vi "FipsAdjacent.vi"() -> (11 "Fips":i32[](array[numeric]))   [LabVIEW 2017] (continued)
TX\"\t48359\t\"Quay County, NM\"\t35037\n\"Oldham County, TX\"\t48359\t\"Deaf Smith County, TX\"\t48117\n\"Oldham County, TX\"\t48359\t\"Hartley County, TX\"\t48205\n\"Oldham County, TX\"\t48359\t\"Moore County, TX\"\t48341\n\"Oldham County, TX\"\t48359\t\"Oldham County, TX\"\t48359\n\"Oldham County, TX\"\t48359\t\"Potter County, TX\"\t48375\n\"Oldham County, TX\"\t48359\t\"Randall County, TX\"\t48381\n\"Orange County, TX\"\t48361\t\"Calcasieu Parish, LA\"\t22019\n\"Orange County, TX\"\t48361\t\"Cameron Parish, LA\"\t22023\n\"Orange County, TX\"\t48361\t\"Hardin County, TX\"\t48199\n\"Orange County, TX\"\t48361\t\"Jasper County, TX\"\t48241\n\"Orange County, TX\"\t48361\t\"Jefferson County, TX\"\t48245\n\"Orange County, TX\"\t48361\t\"Newton County, TX\"\t48351\n\"Orange County, TX\"\t48361\t\"Orange County, TX\"\t48361\n\"Palo Pinto County, TX\"\t48363\t\"Eastland County, TX\"\t48133\n\"Palo Pinto County, TX\"\t48363\t\"Erath County, TX\"\t48143\n\"Palo Pinto County, TX\"\t48363\t\"Hood County, TX\"\t48221\n\"Palo Pinto County, TX\"\t48363\t\"Jack County, TX\"\t48237\n\"Palo Pinto County, TX\"\t48363\t\"Palo Pinto County, TX\"\t48363\n\"Palo Pinto County, TX\"\t48363\t\"Parker County, TX\"\t48367\n\"Palo Pinto County, TX\"\t48363\t\"Stephens County, TX\"\t48429\n\"Palo Pinto County, TX\"\t48363\t\"Young County, TX\"\t48503\n\"Panola County, TX\"\t48365\t\"Caddo Parish, LA\"\t22017\n\"Panola County, TX\"\t48365\t\"De Soto Parish, LA\"\t22031\n\"Panola County, TX\"\t48365\t\"Harrison County, TX\"\t48203\n\"Panola County, TX\"\t48365\t\"Panola County, TX\"\t48365\n\"Panola County, TX\"\t48365\t\"Rusk County, TX\"\t48401\n\"Panola County, TX\"\t48365\t\"Shelby County, TX\"\t48419\n\"Parker County, TX\"\t48367\t\"Hood County, TX\"\t48221\n\"Parker County, TX\"\t48367\t\"Jack County, TX\"\t48237\n\"Parker County, TX\"\t48367\t\"Johnson County, TX\"\t48251\n\"Parker County, TX\"\t48367\t\"Palo Pinto County, TX\"\t48363\n\"Parker County, TX\"\t48367\t\"Parker County, TX\"\t48367\n\"Parker County, TX\"\t48367\t\"Tarrant County, TX\"\t48439\n\"Parker County, TX\"\t48367\t\"Wise County, TX\"\t48497\n\"Parmer County, TX\"\t48369\t\"Curry County, NM\"\t35009\n\"Parmer County, TX\"\t48369\t\"Bailey County, TX\"\t48017\n\"Parmer County, TX\"\t48369\t\"Castro County, TX\"\t48069\n\"Parmer County, TX\"\t48369\t\"Deaf Smith County, TX\"\t48117\n\"Parmer County, TX\"\t48369\t\"Lamb County, TX\"\t48279\n\"Parmer County, TX\"\t48369\t\"Parmer County, TX\"\t48369\n\"Pecos County, TX\"\t48371\t\"Brewster County, TX\"\t48043\n\"Pecos County, TX\"\t48371\t\"Crane County, TX\"\t48103\n\"Pecos County, TX\"\t48371\t\"Crockett County, TX\"\t48105\n\"Pecos County, TX\"\t48371\t\"Jeff Davis County, TX\"\t48243\n\"Pecos County, TX\"\t48371\t\"Pecos County, TX\"\t48371\n\"Pecos County, TX\"\t48371\t\"Reeves County, TX\"\t48389\n\"Pecos County, TX\"\t48371\t\"Terrell County, TX\"\t48443\n\"Pecos County, TX\"\t48371\t\"Ward County, TX\"\t48475\n\"Polk County, TX\"\t48373\t\"Angelina County, TX\"\t48005\n\"Polk County, TX\"\t48373\t\"Hardin County, TX\"\t48199\n\"Polk County, TX\"\t48373\t\"Liberty County, TX\"\t48291\n\"Polk County, TX\"\t48373\t\"Polk County, TX\"\t48373\n\"Polk County, TX\"\t48373\t\"San Jacinto County, TX\"\t48407\n\"Polk County, TX\"\t48373\t\"Trinity County, TX\"\t48455\n\"Polk County, TX\"\t48373\t\"Tyler County, TX\"\t48457\n\"Potter County, TX\"\t48375\t\"Armstrong County, TX\"\t48011\n\"Potter County, TX\"\t48375\t\"Carson County, TX\"\t48065\n\"Potter County, TX\"\t48375\t\"Deaf Smith County, TX\"\t48117\n\"Potter County, TX\"\t48375\t\"Moore County, TX\"\t48341\n\"Potter County, TX\"\t48375\t\"Oldham County, TX\"\t48359\n\"Potter County, TX\"\t48375\t\"Potter County, TX\"\t48375\n\"Potter County, TX\"\t48375\t\"Randall County, TX\"\t48381\n\"Presidio County, TX\"\t48377\t\"Brewster County, TX\"\t48043\n\"Presidio County, TX\"\t48377\t\"Hudspeth County, TX\"\t48229\n\"Presidio County, TX\"\t48377\t\"Jeff Davis County, TX\"\t48243\n\"Presidio County, TX\"\t48377\t\"Presidio County, TX\"\t48377\n\"Rains County, TX\"\t48379\t\"Hopkins County, TX\"\t48223\n\"Rains County, TX\"\t48379\t\"Hunt County, TX\"\t48231\n\"Rains County, TX\"\t48379\t\"Rains County, TX\"\t48379\n\"Rains County, TX\"\t48379\t\"Van Zandt County, TX\"\t48467\n\"Rains County, TX\"\t48379\t\"Wood County, TX\"\t48499\n\"Randall County, TX\"\t48381\t\"Armstrong County, TX\"\t48011\n\"Randall County, TX\"\t48381\t\"Carson County, TX\"\t48065\n\"Randall County, TX\"\t48381\t\"Castro County, TX\"\t48069\n\"Randall County, TX\"\t48381\t\"Deaf Smith County, TX\"\t48117\n\"Randall County, TX\"\t48381\t\"Oldham County, TX\"\t48359\n\"Randall County, TX\"\t48381\t\"Potter County, TX\"\t48375\n\"Randall County, TX\"\t48381\t\"Randall County, TX\"\t48381\n\"Randall County, TX\"\t48381\t\"Swisher County, TX\"\t48437\n\"Reagan County, TX\"\t48383\t\"Crockett County, TX\"\t48105\n\"Reagan County, TX\"\t48383\t\"Glasscock County, TX\"\t48173\n\"Reagan County, TX\"\t48383\t\"Irion County, TX\"\t48235\n\"Reagan County, TX\"\t48383\t\"Midland County, TX\"\t48329\n\"Reagan County, TX\"\t48383\t\"Reagan County, TX\"\t48383\n\"Reagan County, TX\"\t48383\t\"Sterling County, TX\"\t48431\n\"Reagan County, TX\"\t48383\t\"Tom Green County, TX\"\t48451\n\"Reagan County, TX\"\t48383\t\"Upton County, TX\"\t48461\n\"Real County, TX\"\t48385\t\"Bandera County, TX\"\t48019\n\"Real County, TX\"\t48385\t\"Edwards County, TX\"\t48137\n\"Real County, TX\"\t48385\t\"Kerr County, TX\"\t48265\n\"Real County, TX\"\t48385\t\"Real County, TX\"\t48385\n\"Real County, TX\"\t48385\t\"Uvalde County, TX\"\t48463\n\"Red River County, TX\"\t48387\t\"Choctaw County, OK\"\t40023\n\"Red River County, TX\"\t48387\t\"McCurtain County, OK\"\t40089\n\"Red River County, TX\"\t48387\t\"Bowie County, TX\"\t48037\n\"Red River County, TX\"\t48387\t\"Delta County, TX\"\t48119\n\"Red River County, TX\"\t48387\t\"Franklin County, TX\"\t48159\n\"Red River County, TX\"\t48387\t\"Lamar County, TX\"\t48277\n\"Red River County, TX\"\t48387\t\"Morris County, TX\"\t48343\n\"Red River County, TX\"\t48387\t\"Red River County, TX\"\t48387\n\"Red River County, TX\"\t48387\t\"Titus County, TX\"\t48449\n\"Reeves County, TX\"\t48389\t\"Eddy County, NM\"\t35015\n\"Reeves County, TX\"\t48389\t\"Culberson County, TX\"\t48109\n\"Reeves County, TX\"\t48389\t\"Jeff Davis County, TX\"\t48243\n\"Reeves County, TX\"\t48389\t\"Loving County, TX\"\t48301\n\"Reeves County, TX\"\t48389\t\"Pecos County, TX\"\t48371\n\"Reeves County, TX\"\t48389\t\"Reeves County, TX\"\t48389\n\"Reeves County, TX\"\t48389\t\"Ward County, TX\"\t48475\n\"Refugio County, TX\"\t48391\t\"Aransas County, TX\"\t48007\n\"Refugio County, TX\"\t48391\t\"Bee County, TX\"\t48025\n\"Refugio County, TX\"\t48391\t\"Calhoun County, TX\"\t48057\n\"Refugio County, TX\"\t48391\t\"Goliad County, TX\"\t48175\n\"Refugio County, TX\"\t48391\t\"Refugio County, TX\"\t48391\n\"Refugio County, TX\"\t48391\t\"San Patricio County, TX\"\t48409\n\"Refugio County, TX\"\t48391\t\"Victoria County, TX\"\t48469\n\"Roberts County, TX\"\t48393\t\"Carson County, TX\"\t48065\n\"Roberts County, TX\"\t48393\t\"Gray County, TX\"\t48179\n\"Roberts County, TX\"\t48393\t\"Hansford County, TX\"\t48195\n\"Roberts County, TX\"\t48393\t\"Hemphill County, TX\"\t48211\n\"Roberts County, TX\"\t48393\t\"Hutchinson County, TX\"\t48233\n\"Roberts County, TX\"\t48393\t\"Lipscomb County, TX\"\t48295\n\"Roberts County, TX\"\t48393\t\"Ochiltree County, TX\"\t48357\n\"Roberts County, TX\"\t48393\t\"Roberts County, TX\"\t48393\n\"Roberts County, TX\"\t48393\t\"Wheeler County, TX\"\t48483\n\"Robertson County, TX\"\t48395\t\"Brazos County, TX\"\t48041\n\"Robertson County, TX\"\t48395\t\"Burleson County, TX\"\t48051\n\"Robertson County, TX\"\t48395\t\"Falls County, TX\"\t48145\n\"Robertson County, TX\"\t48395\t\"Leon County, TX\"\t48289\n\"Robertson County, TX\"\t48395\t\"Limestone County, TX\"\t48293\n\"Robertson County, TX\"\t48395\t\"Madison County, TX\"\t48313\n\"Robertson County, TX\"\t48395\t\"Milam County, TX\"\t48331\n\"Robertson County, TX\"\t48395\t\"Robertson County, TX\"\t48395\n\"Rockwall County, TX\"\t48397\t\"Collin County, TX\"\t48085\n\"Rockwall County, TX\"\t48397\t\"Dallas County, TX\"\t48113\n\"Rockwall County, TX\"\t48397\t\"Hunt County, TX\"\t48231\n\"Rockwall County, TX\"\t48397\t\"Kaufman County, TX\"\t48257\n\"Rockwall County, TX\"\t48397\t\"Rockwall County, TX\"\t48397\n\"Runnels County, TX\"\t48399\t\"Coke County, TX\"\t48081\n\"Runnels County, TX\"\t48399\t\"Coleman County, TX\"\t48083\n\"Runnels County, TX\"\t48399\t\"Concho County, TX\"\t48095\n\"Runnels County, TX\"\t48399\t\"Nolan County, TX\"\t48353\n\"Runnels County, TX\"\t48399\t\"Runnels County, TX\"\t48399\n\"Runnels County, TX\"\t48399\t\"Taylor County, TX\"\t48441\n\"Runnels County, TX\"\t48399\t\"Tom Green County, TX\"\t48451\n\"Rusk County, TX\"\t48401\t\"Cherokee County, TX\"\t48073\n\"Rusk County, TX\"\t48401\t\"Gregg County, TX\"\t48183\n\"Rusk County, TX\"\t48401\t\"Harrison County, TX\"\t48203\n\"Rusk County, TX\"\t48401\t\"Nacogdoches County, TX\"\t48347\n\"Rusk County, TX\"\t48401\t\"Panola County, TX\"\t48365\n\"Rusk County, TX\"\t48401\t\"Rusk County, TX\"\t48401\n\"Rusk County, TX\"\t48401\t\"Shelby County, TX\"\t48419\n\"Rusk County, TX\"\t48401\t\"Smith County, TX\"\t48423\n\"Sabine County, TX\"\t48403\t\"Sabine Parish, LA\"\t22085\n\"Sabine County, TX\"\t48403\t\"Jasper County, TX\"\t48241\n\"Sabine County, TX\"\t48403\t\"Newton County, TX\"\t48351\n\"Sabine County, TX\"\t48403\t\"Sabine County, TX\"\t48403\n\"Sabine County, TX\"\t48403\t\"San Augustine County, TX\"\t48405\n\"Sabine County, TX\"\t48403\t\"Shelby County, TX\"\t48419\n\"San Augustine County, TX\"\t48405\t\"Angelina County, TX\"\t48005\n\"San Augustine County, TX\"\t48405\t\"Jasper County, TX\"\t48241\n\"San Augustine County, TX\"\t48405\t\"Nacogdoches County, TX\"\t48347\n\"San Augustine County, TX\"\t48405\t\"Sabine County, TX\"\t48403\n\"San Augustine County, TX\"\t48405\t\"San Augustine County, TX\"\t48405\n\"San Augustine County, TX\"\t48405\t\"Shelby County, TX\"\t48419\n\"San Jacinto County, TX\"\t48407\t\"Liberty County, TX\"\t48291\n\"San Jacinto County, TX\"\t48407\t\"Montgomery County, TX\"\t48339\n\"San Jacinto County, TX\"\t48407\t\"Polk County, TX\"\t48373\n\"San Jacinto County, TX\"\t48407\t\"San Jacinto County, TX\"\t48407\n\"San Jacinto County, TX\"\t48407\t\"Trinity County, TX\"\t48455\n\"San Jacinto County, TX\"\t48407\t\"Walker County, TX\"\t48471\n\"San Patricio County, TX\"\t48409\t\"Aransas County, TX\"\t48007\n\"San Patricio County, TX\"\t48409\t\"Bee County, TX\"\t48025\n\"San Patricio County, TX\"\t48409\t\"Jim Wells County, TX\"\t48249\n\"San Patricio County, TX\"\t48409\t\"Live Oak County, TX\"\t48297\n\"San Patricio County, TX\"\t48409\t\"Nueces County, TX\"\t48355\n\"San Patricio County, TX\"\t48409\t\"Refugio County, TX\"\t48391\n\"San Patricio County, TX\"\t48409\t\"San Patricio County, TX\"\t48409\n\"San Saba County, TX\"\t48411\t\"Brown County, TX\"\t48049\n\"San Saba County, TX\"\t48411\t\"Burnet County, TX\"\t48053\n\"San Saba County, TX\"\t48411\t\"Lampasas County, TX\"\t48281\n\"San Saba County, TX\"\t48411\t\"Llano County, TX\"\t48299\n\"San Saba County, TX\"\t48411\t\"McCulloch County, TX\"\t48307\n\"San Saba County, TX\"\t48411\t\"Mason County, TX\"\t48319\n\"San Saba County, TX\"\t48411\t\"Mills County, TX\"\t48333\n\"San Saba County, TX\"\t48411\t\"San Saba County, TX\"\t48411\n\"Schleicher County, TX\"\t48413\t\"Concho County, TX\"\t48095\n\"Schleicher County, TX\"\t48413\t\"Crockett County, TX\"\t48105\n\"Schleicher County, TX\"\t48413\t\"Irion County, TX\"\t48235\n\"Schleicher County, TX\"\t48413\t\"Kimble County, TX\"\t48267\n\"Schleicher County, TX\"\t48413\t\"Menard County, TX\"\t48327\n\"Schleicher County, TX\"\t48413\t\"Schleicher County, TX\"\t48413\n\"Schleicher County, TX\"\t48413\t\"Sutton County, TX\"\t48435\n\"Schleicher County, TX\"\t48413\t\"Tom Green County, TX\"\t48451\n\"Scurry County, TX\"\t48415\t\"Borden County, TX\"\t48033\n\"Scurry County, TX\"\t48415\t\"Fisher County, TX\"\t48151\n\"Scurry County, TX\"\t48415\t\"Garza County, TX\"\t48169\n\"Scurry County, TX\"\t48415\t\"Kent County, TX\"\t48263\n\"Scurry County, TX\"\t48415\t\"Mitchell County, TX\"\t48335\n\"Scurry County, TX\"\t48415\t\"Nolan County, TX\"\t48353\n\"Scurry County, TX\"\t48415\t\"Scurry County, TX\"\t48415\n\"Shackelford County, TX\"\t48417\t\"Callahan County, TX\"\t48059\n\"Shackelford County, TX\"\t48417\t\"Eastland County, TX\"\t48133\n\"Shackelford County, TX\"\t48417\t\"Haskell County, TX\"\t48207\n\"Shackelford County, TX\"\t48417\t\"Jones County, TX\"\t48253\n\"Shackelford County, TX\"\t48417\t\"Shackelford County, TX\"\t48417\n\"Shackelford County, TX\"\t48417\t\"Stephens County, TX\"\t48429\n\"Shackelford County, TX\"\t48417\t\"Throckmorton County, TX\"\t48447\n\"Shelby County, TX\"\t48419\t\"De Soto Parish, LA\"\t22031\n\"Shelby County, TX\"\t48419\t\"Sabine Parish, LA\"\t22085\n\"Shelby County, TX\"\t48419\t\"Nacogdoches County, TX\"\t48347\n\"Shelby County, TX\"\t48419\t\"Panola County, TX\"\t48365\n\"Shelby County, TX\"\t48419\t\"Rusk County, TX\"\t48401\n\"Shelby County, TX\"\t48419\t\"Sabine County, TX\"\t48403\n\"Shelby County, TX\"\t48419\t\"San Augustine County, TX\"\t48405\n\"Shelby County, TX\"\t48419\t\"Shelby County, TX\"\t48419\n\"Sherman County, TX\"\t48421\t\"Cimarron County, OK\"\t40025\n\"Sherman County, TX\"\t48421\t\"Texas County, OK\"\t40139\n\"Sherman County, TX\"\t48421\t\"Dallam County, TX\"\t48111\n\"Sherman County, TX\"\t48421\t\"Hansford County, TX\"\t48195\n\"Sherman County, TX\"\t48421\t\"Hartley County, TX\"\t48205\n\"Sherman County, TX\"\t48421\t\"Hutchinson County, TX\"\t48233\n\"Sherman County, TX\"\t48421\t\"Moore County, TX\"\t48341\n\"Sherman County, TX\"\t48421\t\"Sherman County, TX\"\t48421\n\"Smith County, TX\"\t48423\t\"Cherokee County, TX\"\t48073\n\"Smith County, TX\"\t48423\t\"Gregg County, TX\"\t48183\n\"Smith County, TX\"\t48423\t\"Henderson County, TX\"\t48213\n\"Smith County, TX\"\t48423\t\"Rusk County, TX\"\t48401\n\"Smith County, TX\"\t48423\t\"Smith County, TX\"\t48423\n\"Smith County, TX\"\t48423\t\"Upshur County, TX\"\t48459\n\"Smith County, TX\"\t48423\t\"Van Zandt County, TX\"\t48467\n\"Smith County, TX\"\t48423\t\"Wood County, TX\"\t48499\n\"Somervell County, TX\"\t48425\t\"Bosque County, TX\"\t48035\n\"Somervell County, TX\"\t48425\t\"Erath County, TX\"\t48143\n\"Somervell County, TX\"\t48425\t\"Hood County, TX\"\t48221\n\"Somervell County, TX\"\t48425\t\"Johnson County, TX\"\t48251\n\"Somervell County, TX\"\t48425\t\"Somervell County, TX\"\t48425\n\"Starr County, TX\"\t48427\t\"Brooks County, TX\"\t48047\n\"Starr County, TX\"\t48427\t\"Hidalgo County, TX\"\t48215\n\"Starr County, TX\"\t48427\t\"Jim Hogg County, TX\"\t48247\n\"Starr County, TX\"\t48427\t\"Starr County, TX\"\t48427\n\"Starr County, TX\"\t48427\t\"Zapata County, TX\"\t48505\n\"Stephens County, TX\"\t48429\t\"Eastland County, TX\"\t48133\n\"Stephens County, TX\"\t48429\t\"Palo Pinto County, TX\"\t48363\n\"Stephens County, TX\"\t48429\t\"Shackelford County, TX\"\t48417\n\"Stephens County, TX\"\t48429\t\"Stephens County, TX\"\t48429\n\"Stephens County, TX\"\t48429\t\"Throckmorton County, TX\"\t48447\n\"Stephens County, TX\"\t48429\t\"Young County, TX\"\t48503\n\"Sterling County, TX\"\t48431\t\"Coke County, TX\"\t48081\n\"Sterling County, TX\"\t48431\t\"Glasscock County, TX\"\t48173\n\"Sterling County, TX\"\t48431\t\"Howard County, TX\"\t48227\n\"Sterling County, TX\"\t48431\t\"Mitchell County, TX\"\t48335\n\"Sterling County, TX\"\t48431\t\"Reagan County, TX\"\t48383\n\"Sterling County, TX\"\t48431\t\"Sterling County, TX\"\t48431\n\"Sterling County, TX\"\t48431\t\"Tom Green County, TX\"\t48451\n\"Stonewall County, TX\"\t48433\t\"Dickens County, TX\"\t48125\n\"Stonewall County, TX\"\t48433\t\"Fisher County, TX\"\t48151\n\"Stonewall County, TX\"\t48433\t\"Haskell County, TX\"\t48207\n\"Stonewall County, TX\"\t48433\t\"Jones County, TX\"\t48253\n\"Stonewall County, TX\"\t48433\t\"Kent County, TX\"\t48263\n\"Stonewall County, TX\"\t48433\t\"King County, TX\"\t48269\n\"Stonewall County, TX\"\t48433\t\"Knox County, TX\"\t48275\n\"Stonewall County, TX\"\t48433\t\"Stonewall County, TX\"\t48433\n\"Sutton County, TX\"\t48435\t\"Crockett County, TX\"\t48105\n\"Sutton County, TX\"\t48435\t\"Edwards County, TX\"\t48137\n\"Sutton County, TX\"\t48435\t\"Kimble County, TX\"\t48267\n\"Sutton County, TX\"\t48435\t\"Menard County, TX\"\t48327\n\"Sutton County, TX\"\t48435\t\"Schleicher County, TX\"\t48413\n\"Sutton County, TX\"\t48435\t\"Sutton County, TX\"\t48435\n\"Sutton County, TX\"\t48435\t\"Val Verde County, TX\"\t48465\n\"Swisher County, TX\"\t48437\t\"Armstrong County, TX\"\t48011\n\"Swisher County, TX\"\t48437\t\"Briscoe County, TX\"\t48045\n\"Swisher County, TX\"\t48437\t\"Castro County, TX\"\t48069\n\"Swisher County, TX\"\t48437\t\"Floyd County, TX\"\t48153\n\"Swisher County, TX\"\t48437\t\"Hale County, TX\"\t48189\n\"Swisher County, TX\"\t48437\t\"Randall County, TX\"\t48381\n\"Swisher County, TX\"\t48437\t\"Swisher County, TX\"\t48437\n\"Tarrant County, TX\"\t48439\t\"Dallas County, TX\"\t48113\n\"Tarrant County, TX\"\t48439\t\"Denton County, TX\"\t48121\n\"Tarrant County, TX\"\t48439\t\"Ellis County, TX\"\t48139\n\"Tarrant County, TX\"\t48439\t\"Johnson County, TX\"\t48251\n\"Tarrant County, TX\"\t48439\t\"Parker County, TX\"\t48367\n\"Tarrant County, TX\"\t48439\t\"Tarrant County, TX\"\t48439\n\"Tarrant County, TX\"\t48439\t\"Wise County, TX\"\t48497\n\"Taylor County, TX\"\t48441\t\"Callahan County, TX\"\t48059\n\"Taylor County, TX\"\t48441\t\"Coleman County, TX\"\t48083\n\"Taylor County, TX\"\t48441\t\"Fisher County, TX\"\t48151\n\"Taylor County, TX\"\t48441\t\"Jones County, TX\"\t48253\n\"Taylor County, TX\"\t48441\t\"Nolan County, TX\"\t48353\n\"Taylor County, TX\"\t48441\t\"Runnels County, TX\"\t48399\n\"Taylor County, TX\"\t48441\t\"Taylor County, TX\"\t48441\n\"Terrell County, TX\"\t48443\t\"Brewster County, TX\"\t48043\n\"Terrell County, TX\"\t48443\t\"Crockett County, TX\"\t48105\n\"Terrell County, TX\"\t48443\t\"Pecos County, TX\"\t48371\n\"Terrell County, TX\"\t48443\t\"Terrell County, TX\"\t48443\n\"Terrell County, TX\"\t48443\t\"Val Verde County, TX\"\t48465\n\"Terry County, TX\"\t48445\t\"Cochran County, TX\"\t48079\n\"Terry County, TX\"\t48445\t\"Dawson County, TX\"\t48115\n\"Terry County, TX\"\t48445\t\"Gaines County, TX\"\t48165\n\"Terry County, TX\"\t48445\t\"Hockley County, TX\"\t48219\n\"Terry County, TX\"\t48445\t\"Lubbock County, TX\"\t48303\n\"Terry County, TX\"\t48445\t\"Lynn County, TX\"\t48305\n\"Terry County, TX\"\t48445\t\"Terry County, TX\"\t48445\n\"Terry County, TX\"\t48445\t\"Yoakum County, TX\"\t48501\n\"Throckmorton County, TX\"\t48447\t\"Archer County, TX\"\t48009\n\"Throckmorton County, TX\"\t48447\t\"Baylor County, TX\"\t48023\n\"Throckmorton County, TX\"\t48447\t\"Haskell County, TX\"\t48207\n\"Throckmorton County, TX\"\t48447\t\"Knox County, TX\"\t48275\n\"Throckmorton County, TX\"\t48447\t\"Shackelford County, TX\"\t48417\n\"Throckmorton County, TX\"\t48447\t\"Stephens County, TX\"\t48429\n\"Throckmorton County, TX\"\t48447\t\"Throckmorton County, TX\"\t48447\n\"Throckmorton County, TX\"\t48447\t\"Young County, TX\"\t48503\n\"Titus County, TX\"\t48449\t\"Camp County, TX\"\t48063\n\"Titus County, TX\"\t48449\t\"Franklin County, TX\"\t48159\n\"Titus County, TX\"\t48449\t\"Morris County, TX\"\t48343\n\"Titus County, TX\"\t48449\t\"Red River County, TX\"\t48387\n\"Titus County, TX\"\t48449\t\"Titus County, TX\"\t48449\n\"Tom Green County, TX\"\t48451\t\"Coke County, TX\"\t48081\n\"Tom Green County, TX\"\t48451\t\"Concho County, TX\"\t48095\n\"Tom Green County, TX\"\t48451\t\"Irion County, TX\"\t48235\n\"Tom Green County, TX\"\t48451\t\"Menard County, TX\"\t48327\n\"Tom Green County, TX\"\t48451\t\"Reagan County, TX\"\t48383\n\"Tom Green County, TX\"\t48451\t\"Runnels County, TX\"\t48399\n\"Tom Green County, TX\"\t48451\t\"Schleicher County, TX\"\t48413\n\"Tom Green County, TX\"\t48451\t\"Sterling County, TX\"\t48431\n\"Tom Green County, TX\"\t48451\t\"Tom Green County, TX\"\t48451\n\"Travis County, TX\"\t48453\t\"Bastrop County, TX\"\t48021\n\"Travis County, TX\"\t48453\t\"Blanco County, TX\"\t48031\n\"Travis County, TX\"\t48453\t\"Burnet County, TX\"\t48053\n\"Travis County, TX\"\t48453\t\"Caldwell County, TX\"\t48055\n\"Travis County, TX\"\t48453\t\"Hays County, TX\"\t48209\n\"Travis County, TX\"\t48453\t\"Travis County, TX\"\t48453\n\"Travis County, TX\"\t48453\t\"Williamson County, TX\"\t48491\n\"Trinity County, TX\"\t48455\t\"Angelina County, TX\"\t48005\n\"Trinity County, TX\"\t48455\t\"Houston County, TX\"\t48225\n\"Trinity County, TX\"\t48455\t\"Polk County, TX\"\t48373\n\"Trinity County, TX\"\t48455\t\"San Jacinto County, TX\"\t48407\n\"Trinity County, TX\"\t48455\t\"Trinity County, TX\"\t48455\n\"Trinity County, TX\"\t48455\t\"Walker County, TX\"\t48471\n\"Tyler County, TX\"\t48457\t\"Angelina County, TX\"\t48005\n\"Tyler County, TX\"\t48457\t\"Hardin County, TX\"\t48199\n\"Tyler County, TX\"\t48457\t\"Jasper County, TX\"\t48241\n\"Tyler County, TX\"\t48457\t\"Polk County, TX\"\t48373\n\"Tyler County, TX\"\t48457\t\"Tyler County, TX\"\t48457\n\"Upshur County, TX\"\t48459\t\"Camp County, TX\"\t48063\n\"Upshur County, TX\"\t48459\t\"Gregg County, TX\"\t48183\n\"Upshur County, TX\"\t48459\t\"Harrison County, TX\"\t48203\n\"Upshur County, TX\"\t48459\t\"Marion County, TX\"\t48315\n\"Upshur County, TX\"\t48459\t\"Morris County, TX\"\t48343\n\"Upshur County, TX\"\t48459\t\"Smith County, TX\"\t48423\n\"Upshur County, TX\"\t48459\t\"Upshur County, TX\"\t48459\n\"Upshur County, TX\"\t48459\t\"Wood County, TX\"\t48499\n\"Upton County, TX\"\t48461\t\"Crane County, TX\"\t48103\n\"Upton County, TX\"\t48461\t\"Crockett County, TX\"\t48105\n\"Upton County, TX\"\t48461\t\"Ector County, TX\"\t48135\n\"Upton County, TX\"\t48461\t\"Glasscock County, TX\"\t48173\n\"Upton County, TX\"\t48461\t\"Midland County, TX\"\t48329\n\"Upton County, TX\"\t48461\t\"Reagan County, TX\"\t48383\n\"Upton County, TX\"\t48461\t\"Upton County, TX\"\t48461\n\"Uvalde County, TX\"\t48463\t\"Bandera County, TX\"\t48019\n\"Uvalde County, TX\"\t48463\t\"Edwards County, TX\"\t48137\n\"Uvalde County, TX\"\t48463\t\"Frio County, TX\"\t48163\n\"Uvalde County, TX\"\t48463\t\"Kinney County, TX\"\t48271\n\"Uvalde County, TX\"\t48463\t\"Maverick County, TX\"\t48323\n\"Uvalde County, TX\"\t48463\t\"Medina County, TX\"\t48325\n\"Uvalde County, TX\"\t48463\t\"Real County, TX\"\t48385\n\"Uvalde County, TX\"\t48463\t\"Uvalde County, TX\"\t48463\n\"Uvalde County, TX\"\t48463\t\"Zavala County, TX\"\t48507\n\"Val Verde County, TX\"\t48465\t\"Crockett County, TX\"\t48105\n\"Val Verde County, TX\"\t48465\t\"Edwards County, TX\"\t48137\n\"Val Verde County, TX\"\t48465\t\"Kinney County, TX\"\t48271\n\"Val Verde County, TX\"\t48465\t\"Sutton County, TX\"\t48435\n\"Val Verde County, TX\"\t48465\t\"Terrell County, TX\"\t48443\n\"Val Verde County, TX\"\t48465\t\"Val Verde County, TX\"\t48465\n\"Van Zandt County, TX\"\t48467\t\"Henderson County, TX\"\t48213\n\"Van Zandt County, TX\"\t48467\t\"Hunt County, TX\"\t48231\n\"Van Zandt County, TX\"\t48467\t\"Kaufman County, TX\"\t48257\n\"Van Zandt County, TX\"\t48467\t\"Rains County, TX\"\t48379\n\"Van Zandt County, TX\"\t48467\t\"Smith County, TX\"\t48423\n\"Van Zandt County, TX\"\t48467\t\"Van Zandt County, TX\"\t48467\n\"Van Zandt County, TX\"\t48467\t\"Wood County, TX\"\t48499\n\"Victoria County, TX\"\t48469\t\"Calhoun County, TX\"\t48057\n\"Victoria County, TX\"\t48469\t\"DeWitt County, TX\"\t48123\n\"Victoria County, TX\"\t48469\t\"Goliad County, TX\"\t48175\n\"Victoria County, TX\"\t48469\t\"Jackson County, TX\"\t48239\n\"Victoria County, TX\"\t48469\t\"Lavaca County, TX\"\t48285\n\"Victoria County, TX\"\t48469\t\"Refugio County, TX\"\t48391\n\"Victoria County, TX\"\t48469\t\"Victoria County, TX\"\t48469\n\"Walker County, TX\"\t48471\t\"Grimes County, TX\"\t48185\n\"Walker County, TX\"\t48471\t\"Houston County, TX\"\t48225\n\"Walker County, TX\"\t48471\t\"Madison County, TX\"\t48313\n\"Walker County, TX\"\t48471\t\"Montgomery County, TX\"\t48339\n\"Walker County, TX\"\t48471\t\"San Jacinto County, TX\"\t48407\n\"Walker County, TX\"\t48471\t\"Trinity County, TX\"\t48455\n\"Walker County, TX\"\t48471\t\"Walker County, TX\"\t48471\n\"Waller County, TX\"\t48473\t\"Austin County, TX\"\t48015\n\"Waller County, TX\"\t48473\t\"Fort Bend County, TX\"\t48157\n\"Waller County, TX\"\t48473\t\"Grimes County, TX\"\t48185\n\"Waller County, TX\"\t48473\t\"Harris County, TX\"\t48201\n\"Waller County, TX\"\t48473\t\"Montgomery County, TX\"\t48339\n\"Waller County, TX\"\t48473\t\"Waller County, TX\"\t48473\n\"Waller County, TX\"\t48473\t\"Washington County, TX\"\t48477\n\"Ward County, TX\"\t48475\t\"Crane County, TX\"\t48103\n\"Ward County, TX\"\t48475\t\"Ector County, TX\"\t48135\n\"Ward County, TX\"\t48475\t\"Loving County, TX\"\t48301\n\"Ward County, TX\"\t48475\t\"Pecos County, TX\"\t48371\n\"Ward County, TX\"\t48475\t\"Reeves County, TX\"\t48389\n\"Ward County, TX\"\t48475\t\"Ward County, TX\"\t48475\n\"Ward County, TX\"\t48475\t\"Winkler County, TX\"\t48495\n\"Washington County, TX\"\t48477\t\"Austin County, TX\"\t48015\n\"Washington County, TX\"\t48477\t\"Brazos County, TX\"\t48041\n\"Washington County, TX\"\t48477\t\"Burleson County, TX\"\t48051\n\"Washington County, TX\"\t48477\t\"Fayette County, TX\"\t48149\n\"Washington County, TX\"\t48477\t\"Grimes County, TX\"\t48185\n\"Washington County, TX\"\t48477\t\"Lee County, TX\"\t48287\n\"Washington County, TX\"\t48477\t\"Waller County, TX\"\t48473\n\"Washington County, TX\"\t48477\t\"Washington County, TX\"\t48477\n\"Webb County, TX\"\t48479\t\"Dimmit County, TX\"\t48127\n\"Webb County, TX\"\t48479\t\"Duval County, TX\"\t48131\n\"Webb County, TX\"\t48479\t\"Jim Hogg County, TX\"\t48247\n\"Webb County, TX\"\t48479\t\"La Salle County, TX\"\t48283\n\"Webb County, TX\"\t48479\t\"McMullen County, TX\"\t48311\n\"Webb County, TX\"\t48479\t\"Maverick County, TX\"\t48323\n\"Webb County, TX\"\t48479\t\"Webb County, TX\"\t48479\n\"Webb County, TX\"\t48479\t\"Zapata County, TX\"\t48505\n\"Wharton County, TX\"\t48481\t\"Austin County, TX\"\t48015\n\"Wharton County, TX\"\t48481\t\"Brazoria County, TX\"\t48039\n\"Wharton County, TX\"\t48481\t\"Colorado County, TX\"\t48089\n\"Wharton County, TX\"\t48481\t\"Fort Bend County, TX\"\t48157\n\"Wharton County, TX\"\t48481\t\"Jackson County, TX\"\t48239\n\"Wharton County, TX\"\t48481\t\"Matagorda County, TX\"\t48321\n\"Wharton County, TX\"\t48481\t\"Wharton County, TX\"\t48481\n\"Wheeler County, TX\"\t48483\t\"Beckham County, OK\"\t40009\n\"Wheeler County, TX\"\t48483\t\"Roger Mills County, OK\"\t40129\n\"Wheeler County, TX\"\t48483\t\"Collingsworth County, TX\"\t48087\n\"Wheeler County, TX\"\t48483\t\"Donley County, TX\"\t48129\n\"Wheeler County, TX\"\t48483\t\"Gray County, TX\"\t48179\n\"Wheeler County, TX\"\t48483\t\"Hemphill County, TX\"\t48211\n\"Wheeler County, TX\"\t48483\t\"Roberts County, TX\"\t48393\n\"Wheeler County, TX\"\t48483\t\"Wheeler County, TX\"\t48483\n\"Wichita County, TX\"\t48485\t\"Cotton County, OK\"\t40033\n\"Wichita County, TX\"\t48485\t\"Tillman County, OK\"\t40141\n\"Wichita County, TX\"\t48485\t\"Archer County, TX\"\t48009\n\"Wichita County, TX\"\t48485\t\"Baylor County, TX\"\t48023\n\"Wichita County, TX\"\t48485\t\"Clay County, TX\"\t48077\n\"Wichita County, TX\"\t48485\t\"Wichita County, TX\"\t48485\n\"Wichita County, TX\"\t48485\t\"Wilbarger County, TX\"\t48487\n\"Wilbarger County, TX\"\t48487\t\"Jackson County, OK\"\t40065\n\"Wilbarger County, TX\"\t48487\t\"Tillman County, OK\"\t40141\n\"Wilbarger County, TX\"\t48487\t\"Archer County, TX\"\t48009\n\"Wilbarger County, TX\"\t48487\t\"Baylor County, TX\"\t48023\n\"Wilbarger County, TX\"\t48487\t\"Foard County, TX\"\t48155\n\"Wilbarger County, TX\"\t48487\t\"Hardeman County, TX\"\t48197\n\"Wilbarger County, TX\"\t48487\t\"Wichita County, TX\"\t48485\n\"Wilbarger County, TX\"\t48487\t\"Wilbarger County, TX\"\t48487\n\"Willacy County, TX\"\t48489\t\"Cameron County, TX\"\t48061\n\"Willacy County, TX\"\t48489\t\"Hidalgo County, TX\"\t48215\n\"Willacy County, TX\"\t48489\t\"Kenedy County, TX\"\t48261\n\"Willacy County, TX\"\t48489\t\"Willacy County, TX\"\t48489\n\"Williamson County, TX\"\t48491\t\"Bastrop County, TX\"\t48021\n\"Williamson County, TX\"\t48491\t\"Bell County, TX\"\t48027\n\"Williamson County, TX\"\t48491\t\"Burnet County, TX\"\t48053\n\"Williamson County, TX\"\t48491\t\"Lee County, TX\"\t48287\n\"Williamson County, TX\"\t48491\t\"Milam County, TX\"\t48331\n\"Williamson County, TX\"\t48491\t\"Travis County, TX\"\t48453\n\"Williamson County, TX\"\t48491\t\"Williamson County, TX\"\t48491\n\"Wilson County, TX\"\t48493\t\"Atascosa County, TX\"\t48013\n\"Wilson County, TX\"\t48493\t\"Bexar County, TX\"\t48029\n\"Wilson County, TX\"\t48493\t\"Gonzales County, TX\"\t48177\n\"Wilson County, TX\"\t48493\t\"Guadalupe County, TX\"\t48187\n\"Wilson County, TX\"\t48493\t\"Karnes County, TX\"\t48255\n\"Wilson County, TX\"\t48493\t\"Wilson County, TX\"\t48493\n\"Winkler County, TX\"\t48495\t\"Lea County, NM\"\t35025\n\"Winkler County, TX\"\t48495\t\"Andrews County, TX\"\t48003\n\"Winkler County, TX\"\t48495\t\"Ector County, TX\"\t48135\n\"Winkler County, TX\"\t48495\t\"Loving County, TX\"\t48301\n\"Winkler County, TX\"\t48495\t\"Ward County, TX\"\t48475\n\"Winkler County, TX\"\t48495\t\"Winkler County, TX\"\t48495\n\"Wise County, TX\"\t48497\t\"Cooke County, TX\"\t48097\n\"Wise County, TX\"\t48497\t\"Denton County, TX\"\t48121\n\"Wise County, TX\"\t48497\t\"Jack County, TX\"\t48237\n\"Wise County, TX\"\t48497\t\"Montague County, TX\"\t48337\n\"Wise County, TX\"\t48497\t\"Parker County, TX\"\t48367\n\"Wise County, TX\"\t48497\t\"Tarrant County, TX\"\t48439\n\"Wise County, TX\"\t48497\t\"Wise County, TX\"\t48497\n\"Wood County, TX\"\t48499\t\"Camp County, TX\"\t48063\n\"Wood County, TX\"\t48499\t\"Franklin County, TX\"\t48159\n\"Wood County, TX\"\t48499\t\"Hopkins County, TX\"\t48223\n\"Wood County, TX\"\t48499\t\"Rains County, TX\"\t48379\n\"Wood County, TX\"\t48499\t\"Smith County, TX\"\t48423\n\"Wood County, TX\"\t48499\t\"Upshur County, TX\"\t48459\n\"Wood County, TX\"\t48499\t\"Van Zandt County, TX\"\t48467\n\"Wood County, TX\"\t48499\t\"Wood County, TX\"\t48499\n\"Yoakum County, TX\"\t48501\t\"Lea County, NM\"\t35025\n\"Yoakum County, TX\"\t48501\t\"Cochran County, TX\"\t48079\n\"Yoakum County, TX\"\t48501\t\"Gaines County, TX\"\t48165\n\"Yoakum County, TX\"\t48501\t\"Hockley County, TX\"\t48219\n\"Yoakum County, TX\"\t48501\t\"Terry County, TX\"\t48445\n\"Yoakum County, TX\"\t48501\t\"Yoakum County, TX\"\t48501\n\"Young County, TX\"\t48503\t\"Archer County, TX\"\t48009\n\"Young County, TX\"\t48503\t\"Baylor County, TX\"\t48023\n\"Young County, TX\"\t48503\t\"Jack County, TX\"\t48237\n\"Young County, TX\"\t48503\t\"Palo Pinto County, TX\"\t48363\n\"Young County, TX\"\t48503\t\"Stephens County, TX\"\t48429\n\"Young County, TX\"\t48503\t\"Throckmorton County, TX\"\t48447\n\"Young County, TX\"\t48503\t\"Young County, TX\"\t48503\n\"Zapata County, TX\"\t48505\t\"Jim Hogg County, TX\"\t48247\n\"Zapata County, TX\"\t48505\t\"Starr County, TX\"\t48427\n\"Zapata County, TX\"\t48505\t\"Webb County, TX\"\t48479\n\"Zapata County, TX\"\t48505\t\"Zapata County, TX\"\t48505\n\"Zavala County, TX\"\t48507\t\"Dimmit County, TX\"\t48127\n\"Zavala County, TX\"\t48507\t\"Frio County, TX\"\t48163\n\"Zavala County, TX\"\t48507\t\"Kinney County, TX\"\t48271\n\"Zavala County, TX\"\t48507\t\"Maverick County, TX\"\t48323\n\"Zavala County, TX\"\t48507\t\"Medina County, TX\"\t48325\n\"Zavala County, TX\"\t48507\t\"Uvalde County, TX\"\t48463\n\"Zavala County, TX\"\t48507\t\"Zavala County, TX\"\t48507\n\"Beaver County, UT\"\t49001\t\"Lincoln County, NV\"\t32017\n\"Beaver County, UT\"\t49001\t\"Beaver County, UT\"\t49001\n\"Beaver County, UT\"\t49001\t\"Garfield County, UT\"\t49017\n\"Beaver County, UT\"\t49001\t\"Iron County, UT\"\t49021\n\"Beaver County, UT\"\t49001\t\"Millard County, UT\"\t49027\n\"Beaver County, UT\"\t49001\t\"Piute County, UT\"\t49031\n\"Beaver County, UT\"\t49001\t\"Sevier County, UT\"\t49041\n\"Box Elder County, UT\"\t49003\t\"Cassia County, ID\"\t16031\n\"Box Elder County, UT\"\t49003\t\"Oneida County, ID\"\t16071\n\"Box Elder County, UT\"\t49003\t\"Elko County, NV\"\t32007\n\"Box Elder County, UT\"\t49003\t\"Box Elder County, UT\"\t49003\n\"Box Elder County, UT\"\t49003\t\"Cache County, UT\"\t49005\n\"Box Elder County, UT\"\t49003\t\"Davis County, UT\"\t49011\n\"Box Elder County, UT\"\t49003\t\"Tooele County, UT\"\t49045\n\"Box Elder County, UT\"\t49003\t\"Weber County, UT\"\t49057\n\"Cache County, UT\"\t49005\t\"Bear Lake County, ID\"\t16007\n\"Cache County, UT\"\t49005\t\"Franklin County, ID\"\t16041\n\"Cache County, UT\"\t49005\t\"Oneida County, ID\"\t16071\n\"Cache County, UT\"\t49005\t\"Box Elder County, UT\"\t49003\n\"Cache County, UT\"\t49005\t\"Cache County, UT\"\t49005\n\"Cache County, UT\"\t49005\t\"Rich County, UT\"\t49033\n\"Cache County, UT\"\t49005\t\"Weber County, UT\"\t49057\n\"Carbon County, UT\"\t49007\t\"Carbon County, UT\"\t49007\n\"Carbon County, UT\"\t49007\t\"Duchesne County, UT\"\t49013\n\"Carbon County, UT\"\t49007\t\"Emery County, UT\"\t49015\n\"Carbon County, UT\"\t49007\t\"Sanpete County, UT\"\t49039\n\"Carbon County, UT\"\t49007\t\"Uintah County, UT\"\t49047\n\"Carbon County, UT\"\t49007\t\"Utah County, UT\"\t49049\n\"Daggett County, UT\"\t49009\t\"Moffat County, CO\"\t08081\n\"Daggett County, UT\"\t49009\t\"Daggett County, UT\"\t49009\n\"Daggett County, UT\"\t49009\t\"Duchesne County, UT\"\t49013\n\"Daggett County, UT\"\t49009\t\"Summit County, UT\"\t49043\n\"Daggett County, UT\"\t49009\t\"Uintah County, UT\"\t49047\n\"Daggett County, UT\"\t49009\t\"Sweetwater County, WY\"\t56037\n\"Davis County, UT\"\t49011\t\"Box Elder County, UT\"\t49003\n\"Davis County, UT\"\t49011\t\"Davis County, UT\"\t49011\n\"Davis County, UT\"\t49011\t\"Morgan County, UT\"\t49029\n\"Davis County, UT\"\t49011\t\"Salt Lake County, UT\"\t49035\n\"Davis County, UT\"\t49011\t\"Tooele County, UT\"\t49045\n\"Davis County, UT\"\t49011\t\"Weber County, UT\"\t49057\n\"Duchesne County, UT\"\t49013\t\"Carbon County, UT\"\t49007\n\"Duchesne County, UT\"\t49013\t\"Daggett County, UT\"\t49009\n\"Duchesne County, UT\"\t49013\t\"Duchesne County, UT\"\t49013\n\"Duchesne County, UT\"\t49013\t\"Summit County, UT\"\t49043\n\"Duchesne County, UT\"\t49013\t\"Uintah County, UT\"\t49047\n\"Duchesne County, UT\"\t49013\t\"Utah County, UT\"\t49049\n\"Duchesne County, UT\"\t49013\t\"Wasatch County, UT\"\t49051\n\"Emery County, UT\"\t49015\t\"Carbon County, UT\"\t49007\n\"Emery County, UT\"\t49015\t\"Emery County, UT\"\t49015\n\"Emery County, UT\"\t49015\t\"Grand County, UT\"\t49019\n\"Emery County, UT\"\t49015\t\"San Juan County, UT\"\t49037\n\"Emery County, UT\"\t49015\t\"Sanpete County, UT\"\t49039\n\"Emery County, UT\"\t49015\t\"Sevier County, UT\"\t49041\n\"Emery County, UT\"\t49015\t\"Uintah County, UT\"\t49047\n\"Emery County, UT\"\t49015\t\"Wayne County, UT\"\t49055\n\"Garfield County, UT\"\t49017\t\"Beaver County, UT\"\t49001\n\"Garfield County, UT\"\t49017\t\"Garfield County, UT\"\t49017\n\"Garfield County, UT\"\t49017\t\"Iron County, UT\"\t49021\n\"Garfield County, UT\"\t49017\t\"Kane County, UT\"\t49025\n\"Garfield County, UT\"\t49017\t\"Piute County, UT\"\t49031\n\"Garfield County, UT\"\t49017\t\"San Juan County, UT\"\t49037\n\"Garfield County, UT\"\t49017\t\"Wayne County, UT\"\t49055\n\"Grand County, UT\"\t49019\t\"Garfield County, CO\"\t08045\n\"Grand County, UT\"\t49019\t\"Mesa County, CO\"\t08077\n\"Grand County, UT\"\t49019\t\"Montrose County, CO\"\t08085\n\"Grand County, UT\"\t49019\t\"Emery County, UT\"\t49015\n\"Grand County, UT\"\t49019\t\"Grand County, UT\"\t49019\n\"Grand County, UT\"\t49019\t\"San Juan County, UT\"\t49037\n\"Grand County, UT\"\t49019\t\"Uintah County, UT\"\t49047\n\"Grand County, UT\"\t49019\t\"Wayne County, UT\"\t49055\n\"Iron County, UT\"\t49021\t\"Lincoln County, NV\"\t32017\n\"Iron County, UT\"\t49021\t\"Beaver County, UT\"\t49001\n\"Iron County, UT\"\t49021\t\"Garfield County, UT\"\t49017\n\"Iron County, UT\"\t49021\t\"Iron County, UT\"\t49021\n\"Iron County, UT\"\t49021\t\"Kane County, UT\"\t49025\n\"Iron County, UT\"\t49021\t\"Washington County, UT\"\t49053\n\"Juab County, UT\"\t49023\t\"White Pine County, NV\"\t32033\n\"Juab County, UT\"\t49023\t\"Juab County, UT\"\t49023\n\"Juab County, UT\"\t49023\t\"Millard County, UT\"\t49027\n\"Juab County, UT\"\t49023\t\"Sanpete County, UT\"\t49039\n\"Juab County, UT\"\t49023\t\"Tooele County, UT\"\t49045\n\"Juab County, UT\"\t49023\t\"Utah County, UT\"\t49049\n\"Kane County, UT\"\t49025\t\"Coconino County, AZ\"\t04005\n\"Kane County, UT\"\t49025\t\"Mohave County, AZ\"\t04015\n\"Kane County, UT\"\t49025\t\"Garfield County, UT\"\t49017\n\"Kane County, UT\"\t49025\t\"Iron County, UT\"\t49021\n\"Kane County, UT\"\t49025\t\"Kane County, UT\"\t49025\n\"Kane County, UT\"\t49025\t\"San Juan County, UT\"\t49037\n\"Kane County, UT\"\t49025\t\"Washington County, UT\"\t49053\n\"Millard County, UT\"\t49027\t\"Lincoln County, NV\"\t32017\n\"Millard County, UT\"\t49027\t\"White Pine County, NV\"\t32033\n\"Millard County, UT\"\t49027\t\"Beaver County, UT\"\t49001\n\"Millard County, UT\"\t49027\t\"Juab County, UT\"\t49023\n\"Millard County, UT\"\t49027\t\"Millard County, UT\"\t49027\n\"Millard County, UT\"\t49027\t\"Sanpete County, UT\"\t49039\n\"Millard County, UT\"\t49027\t\"Sevier County, UT\"\t49041\n\"Morgan County, UT\"\t49029\t\"Davis County, UT\"\t49011\n\"Morgan County, UT\"\t49029\t\"Morgan County, UT\"\t49029\n\"Morgan County, UT\"\t49029\t\"Rich County, UT\"\t49033\n\"Morgan County, UT\"\t49029\t\"Salt Lake County, UT\"\t49035\n\"Morgan County, UT\"\t49029\t\"Summit County, UT\"\t49043\n\"Morgan County, UT\"\t49029\t\"Weber County, UT\"\t49057\n\"Piute County, UT\"\t49031\t\"Beaver County, UT\"\t49001\n\"Piute County, UT\"\t49031\t\"Garfield County, UT\"\t49017\n\"Piute County, UT\"\t49031\t\"Piute County, UT\"\t49031\n\"Piute County, UT\"\t49031\t\"Sevier County, UT\"\t49041\n\"Piute County, UT\"\t49031\t\"Wayne County, UT\"\t49055\n\"Rich County, UT\"\t49033\t\"Bear Lake County, ID\"\t16007\n\"Rich County, UT\"\t49033\t\"Franklin County, ID\"\t16041\n\"Rich County, UT\"\t49033\t\"Cache County, UT\"\t49005\n\"Rich County, UT\"\t49033\t\"Morgan County, UT\"\t49029\n\"Rich County, UT\"\t49033\t\"Rich County, UT\"\t49033\n\"Rich County, UT\"\t49033\t\"Summit County, UT\"\t49043\n\"Rich County, UT\"\t49033\t\"Weber County, UT\"\t49057\n\"Rich County, UT\"\t49033\t\"Lincoln County, WY\"\t56023\n\"Rich County, UT\"\t49033\t\"Uinta County, WY\"\t56041\n\"Salt Lake County, UT\"\t49035\t\"Davis County, UT\"\t49011\n\"Salt Lake County, UT\"\t49035\t\"Morgan County, UT\"\t49029\n\"Salt Lake County, UT\"\t49035\t\"Salt Lake County, UT\"\t49035\n\"Salt Lake County, UT\"\t49035\t\"Summit County, UT\"\t49043\n\"Salt Lake County, UT\"\t49035\t\"Tooele County, UT\"\t49045\n\"Salt Lake County, UT\"\t49035\t\"Utah County, UT\"\t49049\n\"Salt Lake County, UT\"\t49035\t\"Wasatch County, UT\"\t49051\n\"San Juan County, UT\"\t49037\t\"Apache County, AZ\"\t04001\n\"San Juan County, UT\"\t49037\t\"Coconino County, AZ\"\t04005\n\"San Juan County, UT\"\t49037\t\"Navajo County, AZ\"\t04017\n\"San Juan County, UT\"\t49037\t\"Dolores County, CO\"\t08033\n\"San Juan County, UT\"\t49037\t\"Mesa County, CO\"\t08077\n\"San Juan County, UT\"\t49037\t\"Montezuma County, CO\"\t08083\n\"San Juan County, UT\"\t49037\t\"Montrose County, CO\"\t08085\n\"San Juan County, UT\"\t49037\t\"San Miguel County, CO\"\t08113\n\"San Juan County, UT\"\t49037\t\"San Juan County, NM\"\t35045\n\"San Juan County, UT\"\t49037\t\"Emery County, UT\"\t49015\n\"San Juan County, UT\"\t49037\t\"Garfield County, UT\"\t49017\n\"San Juan County, UT\"\t49037\t
